vi "GetPulsesFromPulsePositionData.vi"(8 "dt":dbl, 9 "length":i32, 10 "index":i32, 11 "Pulse Positions":T1) -> (1 "count":i32, 2 "pulses":dbl[](array[numeric]))   [LabVIEW 2017, in "DataAccumulator.lvlib"]
uses:
  <vilib>/addons/InsightCM/Devices/Shared/Common/DataAccumulator/DataAccumulator.lvlib
  <vilib>/addons/InsightCM/Utilities/Analysis/Shared/controls/PulsePositions.ctl
  <vilib>/addons/InsightCM/Utilities/Analysis/Shared/AnalysisHelper.lvlib
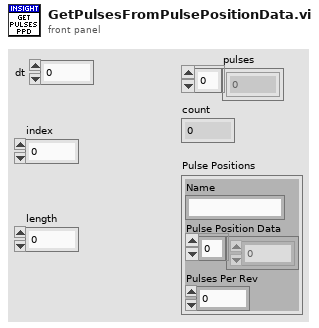
[diagram p1: front panel]
types:
  T1 = typedef "AnalysisHelper.lvlib/PulsePositions.ctl" = cluster{"Name":string, "Pulse Position Data":dbl[], "Pulses Per Rev":i32}
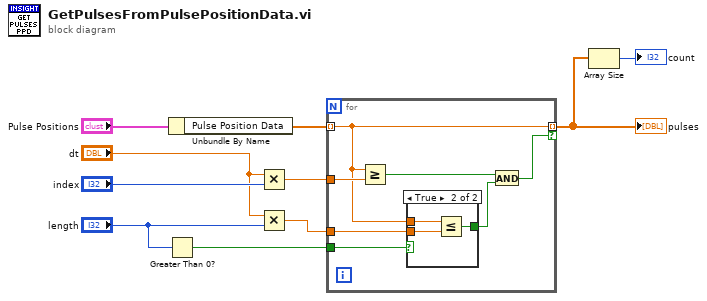
[diagram p0: block diagram]
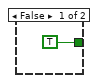
[diagram p2: hidden frame]
diagram:
  n1 = Greater Than 0?(x="length") -> (x > 0?=w5:bool)
  n2 = Unbundle By Name("Pulse Positions") -> ("Pulse Position Data"=w2:dbl[])
  n3 = Multiply(x="dt", y="index") -> (x*y=w8:dbl)
  n4 = Multiply(x="dt", y="length") -> (x*y=w4:dbl)
  n5 = for {
    tunnel: w2 -> [w15] mode=indexing
    tunnel: [w15] -> w7 mode=indexing if=w11
    tunnel: w8 -> [w17]
    tunnel: w5 -> [w16]
    tunnel: w4 -> [w14]
    n6 = Greater Or Equal?(x=w15, y=w17) -> (x >= y?=w12:bool)
    n7 = case shown="True" w16 {
      tunnel: w15 -> [_ w21]
      tunnel: w14 -> [_ w20]
      tunnel: [TRUE w19] -> w13
      frame False {
      }
      frame True {
        n8 = Less Or Equal?(x=w21, y=w20) -> (x <= y?=w19:bool)
      }
    }
    n9 = And(x=w12, y=w13) -> (x .and. y?=w11:bool)
  }
  "pulses" <- w7
  n10 = Array Size(array=w7) -> (size(s)=→"count":i32)
